vi "AMC_QkMvPanSetting.vi"(8 "error in (no error)":errorcluster caption="entrée d'erreur (pas d'erreur)", 11 "Fenêtre face-avant:Limites":T1) -> (0 "error out":errorcluster caption="sortie d'erreur", 3 "Saved set":bool)   [LabVIEW 2019]
uses:
  <vilib>/Utility/miscctls.llb/LVRectTypeDef.ctl
  <vilib>/Utility/config.llb/Read Key (String).vi
  <vilib>/Utility/config.llb/Read Key (U32).vi
  <vilib>/Utility/config.llb/Write Key (String).vi
  <vilib>/Utility/config.llb/Write Key (I32).vi
  <vilib>/Utility/config.llb/NI_LVConfig.lvlib
panel:
  in  "Init":bool
  in  "Save":bool
  in  "Pos3 Name":string
  in  "Pos2 Name":string
  in  "Pos1 Name":string
  in  "Pos3 Axis":enum16{"1", "2", "3"}(ring)
  in  "Pos2 Axis":enum16{"1", "2", "3"}(ring)
  in  "Pos1 Axis":enum16{"1", "2", "3"}(ring)
  in  "Quit":bool
  # "Position1\nLeft/Right"
  # "Position2\nUp/Down"
  # "Position3\nUp/Down"
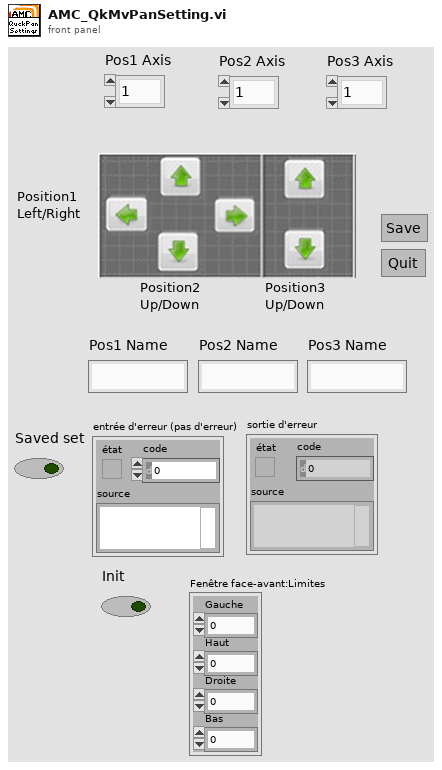
[diagram p1: front panel]
types:
  T1 = typedef "LVRectTypeDef.ctl" = cluster{"Left":i16, "Top":i16, "Right":i16, "Bottom":i16}
  T2 = enum16{"Répertoire du VI actuel", "Répertoire du parent 1", "Répertoire du parent 2", "Répertoire du parent 3"}
  T3 = typedef "NI_LVConfig.lvlib/Config Data RefNum.ctl" = refnum<k1>
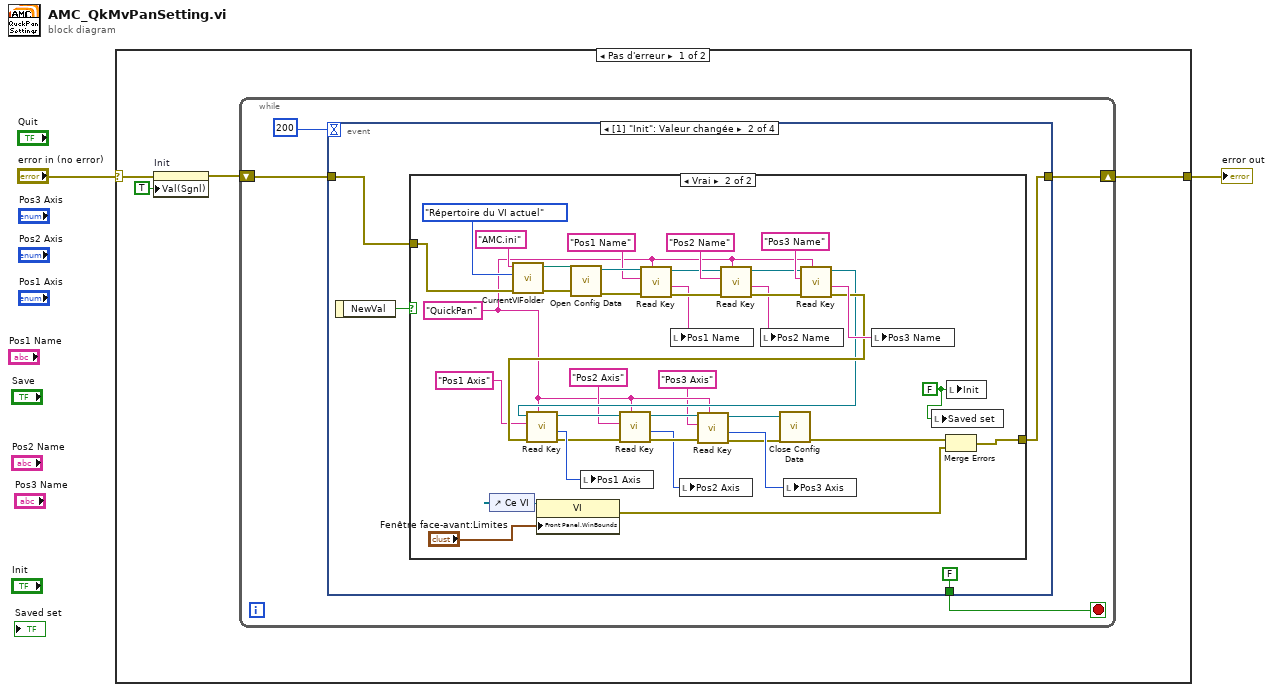
[diagram p0: block diagram]
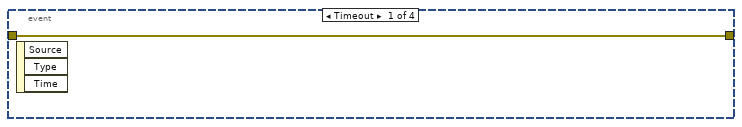
[diagram p2: hidden frame]
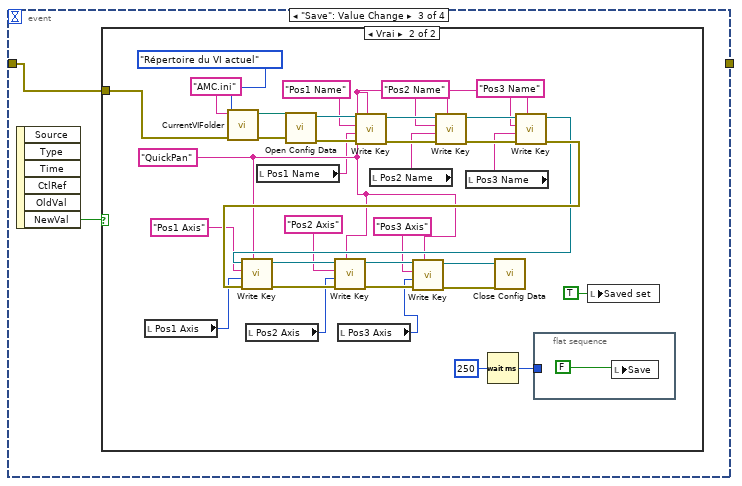
[diagram p4: hidden frame]
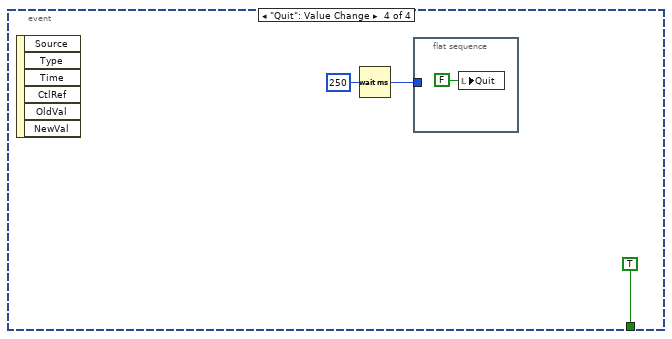
[diagram p6: hidden frame]
diagram:
  n1 = case shown="Pas d'erreur" "error in (no error)" {
    selector: "error in (no error)" -> [w5 w97]
    tunnel: [w6 w97] -> w2
    frame No Error {
      n2 = property on="Init" class="Bool (strict)"(error in=w5, "Val(Sgnl)"=TRUE ("Valeur (Signalisation)")) -> (error out=w4:errorcluster)  [unwired: 1 in, 1 out]
      n3 = while {
        shift-right: [w8] -> w6
        shift-left: w4 -> [w9]
        stop <- w7 stop-if-true
        n4 = event shown="[1] \"Init\": Valeur changée" {
          selector: _ -> [_ _ _ _]
          dyn-events: _ -> [_ _ _ _]
          timeout: 200 -> [_ _ _ _]
          tunnel: w9 -> [w11 w15 w55 _]
          tunnel: [w11 w12 _ _] -> w8
          tunnel: [_ FALSE _ TRUE] -> w7
          event Timeout {
            n5 = event-data() -> ()  [unwired: 1 in, 3 out]
          }
          event "Init": Value Change {
            n6 = event-data() -> ("NewVal"=w14:bool)  [unwired: 1 in]
            n7 = case shown="Vrai" w14 {
              tunnel: w15 -> [w16 w50]
              tunnel: [w16 w20] -> w12
              frame False {
              }
              frame True {
                w21 = FALSE ("Init")
                w28 = "QuickPan" ("section")
                n8 = control-ref of="Ce VI"() -> (w18:refnum<vi>)
                n9 = call <userlib>:"CurrentVIFolder.vi"("error in (no error)"=w50, "Source"=T2."Répertoire du VI actuel", "NomFichier"="AMC.ini") -> ("error out"=w52:errorcluster, "Chemin"=w51:path)  [unwired: 6 in, 1 out]
                n10 = property class="VI"(reference=w18, "Front Panel.WinBounds"="Fenêtre face-avant:Limites") -> (error out=w19:errorcluster)  [unwired: 1 in, 1 out]
                n11 = call <vilib>:"Open Config Data.vi"("error in (no error)"=w52, "configuration file path"=w51) -> ("error out"=w49:errorcluster, "refnum"=w48:T3)  [unwired: 7 in, 1 out]
                n12 = call-poly <vilib>:"Read Key.vi"("section"=w28, "error in (no error)"=w49, "key"="Pos1 Name", "refnum"=w48) -> ("error out"=w46:errorcluster, "value"=w42:string, "refnum out"=w35:T3)  [unwired: 4 in, 1 out]
                n13 = local write "Pos1 Name"(w42) -> ()
                n14 = call-poly <vilib>:"Read Key.vi"("section"=w28, "error in (no error)"=w46, "key"="Pos2 Name", "refnum"=w35) -> ("error out"=w45:errorcluster, "value"=w41:string, "refnum out"=w34:T3)  [unwired: 4 in, 1 out]
                n15 = local write "Pos2 Name"(w41) -> ()
                n16 = call-poly <vilib>:"Read Key.vi"("section"=w28, "error in (no error)"=w45, "key"="Pos3 Name", "refnum"=w34) -> ("error out"=w39:errorcluster, "value"=w40:string, "refnum out"=w33:T3)  [unwired: 4 in, 1 out]
                n17 = call-poly <vilib>:"Read Key.vi"("section"=w28, "error in (no error)"=w39, "key"="Pos1 Axis", "refnum"=w33) -> ("error out"=w36:errorcluster, "value"=w37:u32, "refnum out"=w32:T3)  [unwired: 4 in, 1 out]
                n18 = local write "Pos1 Axis"(w37) -> ()
                n19 = call-poly <vilib>:"Read Key.vi"("section"=w28, "error in (no error)"=w36, "key"="Pos2 Axis", "refnum"=w32) -> ("error out"=w30:errorcluster, "value"=w27:u32, "refnum out"=w29:T3)  [unwired: 4 in, 1 out]
                n20 = local write "Pos2 Axis"(w27) -> ()
                n21 = call-poly <vilib>:"Read Key.vi"("section"=w28, "error in (no error)"=w30, "key"="Pos3 Axis", "refnum"=w29) -> ("error out"=w24:errorcluster, "value"=w26:u32, "refnum out"=w23:T3)  [unwired: 4 in, 1 out]
                n22 = call <vilib>:"Close Config Data.vi"("error in (no error)"=w24, "refnum"=w23) -> ("error out"=w22:errorcluster)  [unwired: 8 in, 1 out]
                n23 = local write "Pos3 Axis"(w26) -> ()
                n24 = local write "Pos3 Name"(w40) -> ()
                n25 = local write "Saved set"(w21) -> ()
                n26 = Merge Errors(w22, w19) -> (w20:errorcluster)
                n27 = local write "Init"(w21) -> ()
              }
            }
          }
          event "Save": Value Change {
            n28 = event-data() -> ("NewVal"=w56:bool)  [unwired: 1 in, 5 out]
            n29 = case shown="Vrai" w56 {
              tunnel: w55 -> [_ w64]
              frame False {
              }
              frame True {
                w73 = "QuickPan" ("section")
                n30 = local read "Pos1 Axis"() -> (w60:enum16{"1", "2", "3"})
                n31 = call <userlib>:"CurrentVIFolder.vi"("error in (no error)"=w64, "Source"=T2."Répertoire du VI actuel", "NomFichier"="AMC.ini") -> ("error out"=w89:errorcluster, "Chemin"=w88:path)  [unwired: 6 in, 1 out]
                n32 = local read "Pos2 Axis"() -> (w59:enum16{"1", "2", "3"})
                n33 = local read "Pos1 Name"() -> (w63:string)
                n34 = call <vilib>:"Open Config Data.vi"("error in (no error)"=w89, "configuration file path"=w88) -> ("error out"=w87:errorcluster, "refnum"=w86:T3)  [unwired: 7 in, 1 out]
                n35 = local read "Pos3 Axis"() -> (w58:enum16{"1", "2", "3"})
                n36 = call-poly <vilib>:"Write Key.vi"("section"=w73, "error in (no error)"=w87, "value"=w63, "key"="Pos1 Name", "refnum"=w86) -> ("error out"=w85:errorcluster, "refnum out"=w81:T3)  [unwired: 4 in, 1 out]
                n37 = local read "Pos2 Name"() -> (w62:string)
                n38 = call-poly <vilib>:"Write Key.vi"("section"=w73, "error in (no error)"=w85, "value"=w62, "key"="Pos2 Name", "refnum"=w81) -> ("error out"=w84:errorcluster, "refnum out"=w80:T3)  [unwired: 4 in, 1 out]
                n39 = local read "Pos3 Name"() -> (w61:string)
                n40 = Wait (ms)(milliseconds to wait=u32 250 ("attente (ms)")) -> (millisecond timer value=w91:u32)
                n41 = call-poly <vilib>:"Write Key.vi"("section"=w73, "error in (no error)"=w84, "value"=w61, "key"="Pos3 Name", "refnum"=w80) -> ("error out"=w83:errorcluster, "refnum out"=w79:T3)  [unwired: 4 in, 1 out]
                n42 = call-poly <vilib>:"Write Key.vi"("section"=w73, "error in (no error)"=w83, "value"=w60, "key"="Pos1 Axis", "refnum"=w79) -> ("error out"=w82:errorcluster, "refnum out"=w78:T3)  [unwired: 4 in, 1 out]
                n43 = call-poly <vilib>:"Write Key.vi"("section"=w73, "error in (no error)"=w82, "value"=w59, "key"="Pos2 Axis", "refnum"=w78) -> ("error out"=w77:errorcluster, "refnum out"=w76:T3)  [unwired: 4 in, 1 out]
                n44 = call-poly <vilib>:"Write Key.vi"("section"=w73, "error in (no error)"=w77, "value"=w58, "key"="Pos3 Axis", "refnum"=w76) -> ("error out"=w75:errorcluster, "refnum out"=w74:T3)  [unwired: 4 in, 1 out]
                n45 = call <vilib>:"Close Config Data.vi"("error in (no error)"=w75, "refnum"=w74) -> ()  [unwired: 8 in, 2 out]
                n46 = flat-sequence {
                  tunnel: w91 -> [_]
                  frame #0 {
                    n47 = local write "Save"(FALSE ("Save")) -> ()
                  }
                }
                n48 = local write "Saved set"(TRUE ("Saved set")) -> ()
              }
            }
          }
          event "Quit": Value Change {
            n49 = event-data() -> ()  [unwired: 1 in, 6 out]
            n50 = Wait (ms)(milliseconds to wait=u32 250 ("attente (ms)")) -> (millisecond timer value=w94:u32)
            n51 = flat-sequence {
              tunnel: w94 -> [_]
              frame #0 {
                n52 = local write "Quit"(FALSE ("Quit")) -> ()
              }
            }
          }
        }
      }
    }
    frame Error {
    }
  }
  "error out" <- w2
